vi "Extract First Quoted String.vi"(9 "Strip Quotes (FALSE)":bool, 11 "Quoted String":string) -> (1 "offset past match":i32, 2 "After First Quoted String":string, 3 "First Quoted String":string)   [LabVIEW 2020, in "jki_python_data_tools.lvlib"]
uses:
  jki_python_data_tools.lvlib
panel:
  # "Copyright © 2003-2009 JKI. All rights reserved.\n\nAuthor: Jim Kring [jim.kring@jameskring.com]\n\nThis library is provided \"AS IS\" ,WITHOUT WARRANTIES OR \nCONDITIONS OF ANY KIND, either express or implied.\n\nJames Kring, Inc. -- http://www.jameskring.com"
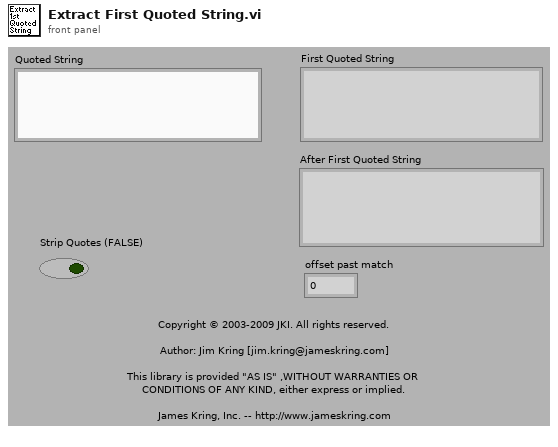
[diagram p1: front panel]
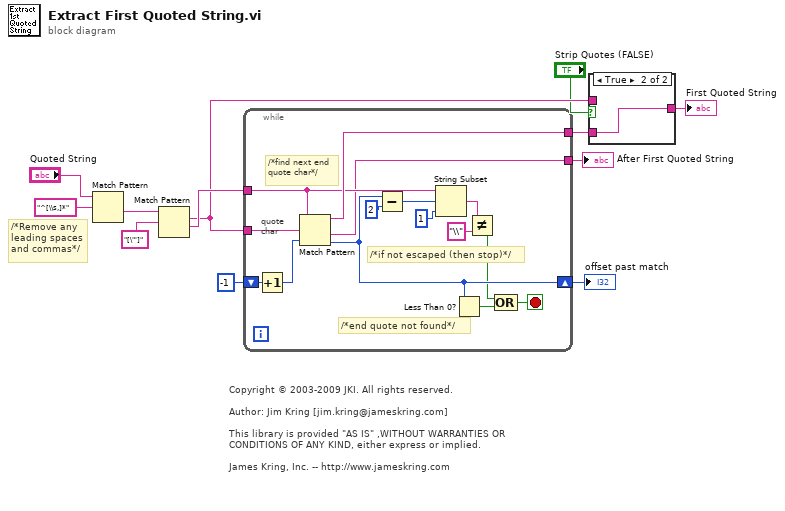
[diagram p0: block diagram]
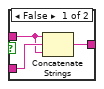
[diagram p2: hidden frame]
diagram:
  # "Copyright © 2003-2009 JKI. All rights reserved.\n\nAuthor: Jim Kring [jim.kring@jameskring.com]\n\nThis library is provided \"AS IS\" ,WITHOUT WARRANTIES OR \nCONDITIONS OF ANY KIND, either express or implied.\n\nJames Kring, Inc. -- http://www.jameskring.com"
  # "/*Remove any leading spaces and commas*/"
  n1 = Match Pattern(string="Quoted String", regular expression="^[\\s,]*") -> (after substring=w8:string)  [unwired: 1 in, 3 out]
  n2 = Match Pattern(string=w8, regular expression="[\"']" ("search string/char (-)")) -> (match substring=w2:string, after substring=w6:string)  [unwired: 1 in, 2 out]
  n3 = while {
    tunnel: w6 -> [w15]
    shift-right: [w23] -> w12
    shift-left: -1 ("offset past match") -> [w27]
    tunnel: w2 -> [w26]
    tunnel: [w16] -> w3
    tunnel: [w13] -> w11
    stop <- w24 stop-if-true
    # "/*find next end quote char*/"
    # "/*end quote not found*/"
    # "/*if not escaped (then stop)*/"
    # "quote char"
    n4 = Increment(x=w27) -> (x+1=w14:i32)
    n5 = Match Pattern(string=w15, regular expression=w26, offset (0)=w14) -> (before substring=w16:string, after substring=w13:string, offset past match=w23:i32)  [unwired: 1 out]
    n6 = Subtract(x=w23, y=2) -> (x-y=w21:i32)
    n7 = String Subset(string=w15, offset (0)=w21, length (rest)=1 ("length (rest)")) -> (substring=w19:string)
    n8 = Less Than 0?(x=w23) -> (x < 0?=w25:bool)
    n9 = Not Equal?(x=w19, y="\\" ("x")) -> (x != y?=w17:bool)
    n10 = Compound Arithmetic op=OR(w17, w25) -> (w24:bool)
  }
  "offset past match" <- w12
  "After First Quoted String" <- w11
  n11 = case shown="True" "Strip Quotes (FALSE)" {
    tunnel: [w30 w31] -> w4
    tunnel: w3 -> [w29 w31]
    tunnel: w2 -> [w28 _]
    frame False {
      n12 = Concatenate Strings(w28, w29, w28) -> (w30:string)
    }
    frame True {
    }
  }
  "First Quoted String" <- w4
